vi "Write all Set Messages.vi"(11 "Device Communication and Control Abstract In":refnum<class "Device Communication and Control Abstract.lvclass">) -> (3 "Device Communication and Control Abstract Out":refnum<class "Device Communication and Control Abstract.lvclass">)   [LabVIEW 2018, in "EMS Core.lvlib" / "EMS.lvclass"]
doc: "Given that all Optimazation Actors could possibly need access to all control messages for IEDs, a single subVI provides this function to all optimization launchers."
uses:
  EMS.lvclass
  Device Communication and Control Abstract Actor/Device Communication and Control Abstract/Device Communication and Control Abstract.lvclass
  C:/Users/Administrator/Desktop/LabVIEW EMS/EMS Generic Actor/EMS Generic/EMS Generic.lvclass
  EMS Messages/DER Control Msg/DER Control Msg.lvclass
  C:/Users/Administrator/Desktop/LabVIEW EMS/Device Communication and Control Abstract Actor/Device Communication and Control Abstract Messages/Set DER Control Msg/Set DER Control Msg.lvclass
  EMS Messages/DER setGenerationMode Msg/DER setGenerationMode Msg.lvclass
  C:/Users/Administrator/Desktop/LabVIEW EMS/Device Communication and Control Abstract Actor/Device Communication and Control Abstract Messages/Set DER GenerationMode Msg/Set DER GenerationMode Msg.lvclass
  EMS Messages/DER SetpointP Msg/DER SetpointP Msg.lvclass
  C:/Users/Administrator/Desktop/LabVIEW EMS/Device Communication and Control Abstract Actor/Device Communication and Control Abstract Messages/Set DER SetPointP Msg/Set DER SetPointP Msg.lvclass
  EMS Messages/DER SetpointPF Msg/DER SetpointPF Msg.lvclass
  C:/Users/Administrator/Desktop/LabVIEW EMS/Device Communication and Control Abstract Actor/Device Communication and Control Abstract Messages/Set DER SetPointPF Msg/Set DER SetPointPF Msg.lvclass
  EMS Messages/DER SetpointQ Msg/DER SetpointQ Msg.lvclass
  C:/Users/Administrator/Desktop/LabVIEW EMS/Device Communication and Control Abstract Actor/Device Communication and Control Abstract Messages/Set DER SetPointQ Msg/Set DER SetPointQ Msg.lvclass
  EMS Messages/DER SetpointV Msg/DER SetpointV Msg.lvclass
  C:/Users/Administrator/Desktop/LabVIEW EMS/Device Communication and Control Abstract Actor/Device Communication and Control Abstract Messages/Set DER SetPointV Msg/Set DER SetPointV Msg.lvclass
  EMS Messages/DER VF Msg/DER VF Msg.lvclass
  C:/Users/Administrator/Desktop/LabVIEW EMS/Device Communication and Control Abstract Actor/Device Communication and Control Abstract Messages/Set DER VF Msg/Set DER VF Msg.lvclass
  EMS Messages/HVAC Control Msg/HVAC Control Msg.lvclass
  C:/Users/Administrator/Desktop/LabVIEW EMS/Device Communication and Control Abstract Actor/Device Communication and Control Abstract Messages/Set HVAC Control Msg/Set HVAC Control Msg.lvclass
  EMS Messages/IED setMicrogridID Msg/IED setMicrogridID Msg.lvclass
  C:/Users/Administrator/Desktop/LabVIEW EMS/Device Communication and Control Abstract Actor/Device Communication and Control Abstract Messages/Set IED MicrogridID Msg/Set IED MicrogridID Msg.lvclass
  EMS Messages/Load Control Msg/Load Control Msg.lvclass
  C:/Users/Administrator/Desktop/LabVIEW EMS/Device Communication and Control Abstract Actor/Device Communication and Control Abstract Messages/Set Load Control Msg/Set Load Control Msg.lvclass
  EMS Messages/PCC Transition Msg/PCC Transition Msg.lvclass
  C:/Users/Administrator/Desktop/LabVIEW EMS/Device Communication and Control Abstract Actor/Device Communication and Control Abstract Messages/Set PCC Transition Msg/Set PCC Transition Msg.lvclass
  EMS Messages/Relay Control Msg/Relay Control Msg.lvclass
  C:/Users/Administrator/Desktop/LabVIEW EMS/Device Communication and Control Abstract Actor/Device Communication and Control Abstract Messages/Set Relay Control Msg/Set Relay Control Msg.lvclass
  EMS Messages/IED watchdogReset Msg/IED watchdogReset Msg.lvclass
  C:/Users/Administrator/Desktop/LabVIEW EMS/Device Communication and Control Abstract Actor/Device Communication and Control Abstract Messages/Set IED watchdogReset Msg/Set IED watchdogReset Msg.lvclass
  EMS Messages/DER SetpointF Msg/DER SetpointF Msg.lvclass
  C:/Users/Administrator/Desktop/LabVIEW EMS/Device Communication and Control Abstract Actor/Device Communication and Control Abstract Messages/Set DER SetPointF Msg/Set DER SetPointF Msg.lvclass
  EMS Messages/IED setMicrogridID (Single) Msg/IED setMicrogridID (Single) Msg.lvclass
  C:/Users/Administrator/Desktop/LabVIEW EMS/Device Communication and Control Abstract Actor/Device Communication and Control Abstract Messages/Set Single Device IED MicrogridID Msg/Set Single Device IED MicrogridID Msg.lvclass
  EMS Messages/ForecastData Long Msg/ForecastData Long Msg.lvclass
  C:/Users/Administrator/Desktop/LabVIEW EMS/Device Communication and Control Abstract Actor/Device Communication and Control Abstract Messages/Set ForecastData Long Msg/Set ForecastData Long Msg.lvclass
  EMS Messages/Pass Through Device State Information Msg/Pass Through Device State Information Msg.lvclass
  C:/Users/Administrator/Desktop/LabVIEW EMS/EMS Generic Actor/EMS Generic Messages/Device State Information Msg/Device State Information Msg.lvclass
  EMS Messages/Pass Through Current Status Msg/Pass Through Current Status Msg.lvclass
  C:/Users/Administrator/Desktop/LabVIEW EMS/EMS Generic Actor/EMS Generic Messages/Return String Msg/Return String Msg.lvclass
  Device Communication and Control Abstract Actor/Device Communication and Control Abstract/Device Communication and Control Abstract.lvclass/Device Communication and Control Abstract.ctl
  EMS Generic Actor/EMS Generic/EMS Generic.lvclass/EMS Generic.ctl
  EMS Generic Actor/EMS Generic/EMS Generic.lvclass
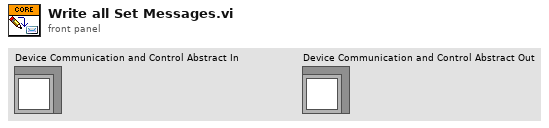
[diagram p1: front panel]
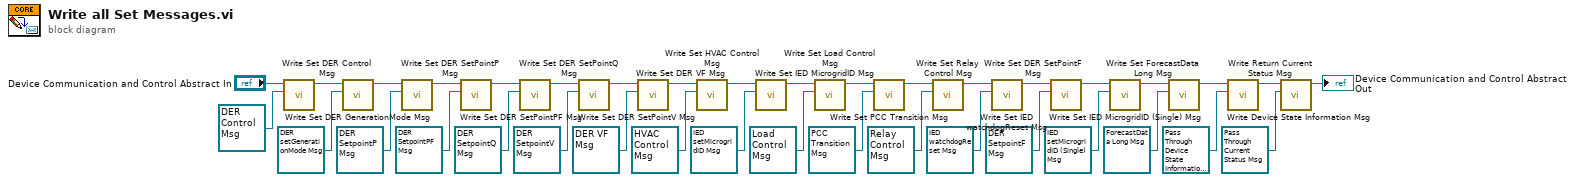
[diagram p0: block diagram]
diagram:
  n1 = call "Write Set DER Control Msg.vi"("Set DER Control Msg"=refnum<class "DER Control Msg.lvclass"> refnum ("SCADA Core.lvlib:DER Control Msg.lvclass"), "SCADA Sub Abstract in"="Device Communication and Control Abstract In") -> ("SCADA Sub Abstract out"=w36:refnum<class "Device Communication and Control Abstract.lvclass">)  [unwired: 9 in]
  n2 = call "Write Set DER GenerationMode Msg.vi"("Set DER GenerationMode Msg"=refnum<class "DER setGenerationMode Msg.lvclass"> refnum ("SCADA Core.lvlib:DER setGenerationMode Msg.lvclass"), "SCADA Sub Abstract in"=w36) -> ("SCADA Sub Abstract out"=w35:refnum<class "Device Communication and Control Abstract.lvclass">)  [unwired: 9 in]
  n3 = call "Write Set DER SetPointP Msg.vi"("Set DER SetPointP Msg"=refnum<class "DER SetpointP Msg.lvclass"> refnum ("SCADA Core.lvlib:DER SetpointP Msg.lvclass"), "SCADA Sub Abstract in"=w35) -> ("SCADA Sub Abstract out"=w34:refnum<class "Device Communication and Control Abstract.lvclass">)  [unwired: 9 in]
  n4 = call "Write Set DER SetPointPF Msg.vi"("Set DER SetPointPF Msg"=refnum<class "DER SetpointPF Msg.lvclass"> refnum ("SCADA Core.lvlib:DER SetpointPF Msg.lvclass"), "SCADA Sub Abstract in"=w34) -> ("SCADA Sub Abstract out"=w33:refnum<class "Device Communication and Control Abstract.lvclass">)  [unwired: 9 in]
  n5 = call "Write Set DER SetPointQ Msg.vi"("Set DER SetPointQ Msg"=refnum<class "DER SetpointQ Msg.lvclass"> refnum ("SCADA Core.lvlib:DER SetpointQ Msg.lvclass"), "SCADA Sub Abstract in"=w33) -> ("SCADA Sub Abstract out"=w32:refnum<class "Device Communication and Control Abstract.lvclass">)  [unwired: 9 in]
  n6 = call "Write Set DER SetPointV Msg.vi"("Set DER SetPointV Msg"=refnum<class "DER SetpointV Msg.lvclass"> refnum ("SCADA Core.lvlib:DER SetpointVF Msg.lvclass"), "SCADA Sub Abstract in"=w32) -> ("SCADA Sub Abstract out"=w31:refnum<class "Device Communication and Control Abstract.lvclass">)  [unwired: 9 in]
  n7 = call "Write Set DER VF Msg.vi"("Set DER VF Msg"=refnum<class "DER VF Msg.lvclass"> refnum ("SCADA Core.lvlib:DER VF Msg.lvclass"), "SCADA Sub Abstract in"=w31) -> ("SCADA Sub Abstract out"=w30:refnum<class "Device Communication and Control Abstract.lvclass">)  [unwired: 9 in]
  n8 = call "Write Set HVAC Control Msg.vi"("Set HVAC Control Msg"=refnum<class "HVAC Control Msg.lvclass"> refnum ("SCADA Core.lvlib:HVAC Control Msg.lvclass"), "SCADA Sub Abstract in"=w30) -> ("SCADA Sub Abstract out"=w29:refnum<class "Device Communication and Control Abstract.lvclass">)  [unwired: 9 in]
  n9 = call "Write Set IED MicrogridID Msg.vi"("Set IED MicrogridID Msg"=refnum<class "IED setMicrogridID Msg.lvclass"> refnum ("SCADA Core.lvlib:IED setMicrogridID Msg.lvclass"), "SCADA Sub Abstract in"=w29) -> ("SCADA Sub Abstract out"=w28:refnum<class "Device Communication and Control Abstract.lvclass">)  [unwired: 9 in]
  n10 = call "Write Set Load Control Msg.vi"("Set Load Control Msg"=refnum<class "Load Control Msg.lvclass"> refnum ("SCADA Core.lvlib:Load Control Msg.lvclass"), "SCADA Sub Abstract in"=w28) -> ("SCADA Sub Abstract out"=w27:refnum<class "Device Communication and Control Abstract.lvclass">)  [unwired: 9 in]
  n11 = call "Write Set PCC Transition Msg.vi"("Set PCC Transition Msg"=refnum<class "PCC Transition Msg.lvclass"> refnum ("SCADA Core.lvlib:PCC Transition Msg.lvclass"), "SCADA Sub Abstract in"=w27) -> ("SCADA Sub Abstract out"=w26:refnum<class "Device Communication and Control Abstract.lvclass">)  [unwired: 9 in]
  n12 = call "Write Set Relay Control Msg.vi"("Set Relay Control Msg"=refnum<class "Relay Control Msg.lvclass"> refnum ("SCADA Core.lvlib:Relay Control Msg.lvclass"), "SCADA Sub Abstract in"=w26) -> ("SCADA Sub Abstract out"=w12:refnum<class "Device Communication and Control Abstract.lvclass">)  [unwired: 9 in]
  n13 = call "Write Set IED watchdogReset Msg.vi"("Set IED watchdogReset Msg"=refnum<class "IED watchdogReset Msg.lvclass"> refnum ("SCADA Core.lvlib:IED watchdogReset Msg.lvclass"), "SCADA Sub Abstract in"=w12) -> ("SCADA Sub Abstract out"=w11:refnum<class "Device Communication and Control Abstract.lvclass">)  [unwired: 9 in]
  n14 = call "Write Set DER SetPointF Msg.vi"("Set DER SetPointF Msg"=refnum<class "DER SetpointF Msg.lvclass"> refnum ("SCADA Core.lvlib:DER SetpointF Msg.lvclass"), "SCADA Sub Abstract in"=w11) -> ("SCADA Sub Abstract out"=w9:refnum<class "Device Communication and Control Abstract.lvclass">)  [unwired: 9 in]
  n15 = call "Write Set IED MicrogridID (Single) Msg.vi"("Set IED MicrogridID (Single) Msg"=refnum<class "IED setMicrogridID (Single) Msg.lvclass"> refnum ("SCADA Core.lvlib:IED setMicrogridID (Single) Msg.lvclass"), "SCADA Sub Abstract in"=w9) -> ("SCADA Sub Abstract out"=w7:refnum<class "Device Communication and Control Abstract.lvclass">)  [unwired: 9 in]
  n16 = call "Write Set ForecastData Long Msg.vi"("Set ForecastData Long Msg"=refnum<class "ForecastData Long Msg.lvclass"> refnum ("SCADA Core.lvlib:ForecastData Long Msg.lvclass"), "SCADA Sub Abstract in"=w7) -> ("SCADA Sub Abstract out"=w5:refnum<class "Device Communication and Control Abstract.lvclass">)  [unwired: 9 in]
  n17 = call "Write Device State Information Msg.vi"("Device State Information Msg"=refnum<class "Pass Through Device State Information Msg.lvclass"> refnum ("EMS Core.lvlib:Pass Through Device State Information Msg.lvclass"), "EMS Generic in"=w5) -> ("EMS Generic out"=w3:refnum<class "Device Communication and Control Abstract.lvclass">)  [unwired: 9 in]
  n18 = call "Write Return Current Status Msg.vi"("EMS Generic Actor.lvlib:Return String Msg.lvclass"=refnum<class "Pass Through Current Status Msg.lvclass"> refnum ("EMS Core.lvlib:Pass Through Current Status Msg.lvclass"), "EMS Generic in"=w3) -> ("EMS Generic out"=→"Device Communication and Control Abstract Out":refnum<class "Device Communication and Control Abstract.lvclass">)  [unwired: 9 in]
